vi "Increment Timer.vi"(8 "error in (no error)":errorcluster, 11 "Timer in":refnum<class "Timer.lvclass">) -> (0 "error out":errorcluster, 3 "Timer out":refnum<class "Timer.lvclass">)   [LabVIEW 2024, in "Timer.lvlib" / "Timer.lvclass"]
uses:
  Timer.lvclass
  Applications/National Instruments/LabVIEW 2024 64-bit/vi.lib/ActorFramework/Actor/Actor.lvclass
  Timer.lvclass/Timer.ctl
  <vilib>/ActorFramework/Actor/Actor.lvclass/Actor.ctl
  <vilib>/ActorFramework/Message Enqueuer/Message Enqueuer.lvclass/Message Enqueuer.ctl
  <vilib>/ActorFramework/Message Enqueuer/Init from Existing Queue.vi
  <vilib>/ActorFramework/Message Enqueuer/Enqueue.vi
  Timer Messages/Publish Updates Msg/Publish Updates Msg.lvclass
  Applications/National Instruments/LabVIEW 2024 64-bit/vi.lib/ActorFramework/Message/Message.lvclass
  Timer Messages/Stop Timer Msg/Stop Timer Msg.lvclass
  Timer Messages/Increment Timer Msg/Increment Timer Msg.lvclass
  <vilib>/ActorFramework/Message Priority Queue/Priority Enqueue.vi
  <vilib>/ActorFramework/Message Enqueuer/Message Enqueuer.lvclass
  <vilib>/ActorFramework/Actor/Actor.lvclass
  Users/elijahkerry/challenge-of-champions/Timer/Timer/Timer.lvclass
panel:
  out "x-y":dbl format="%#_6f"
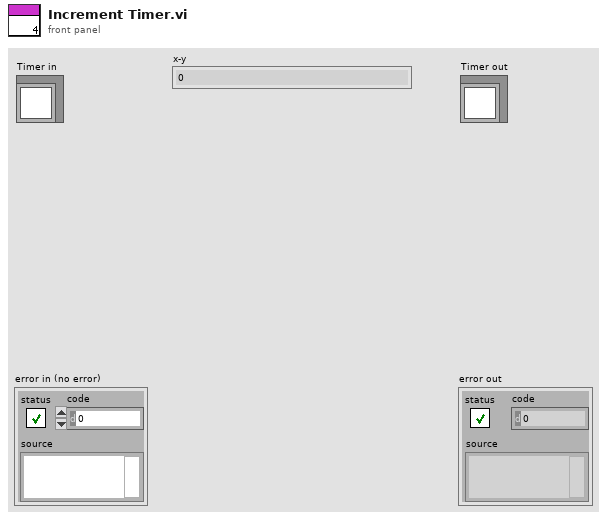
[diagram p1: front panel]
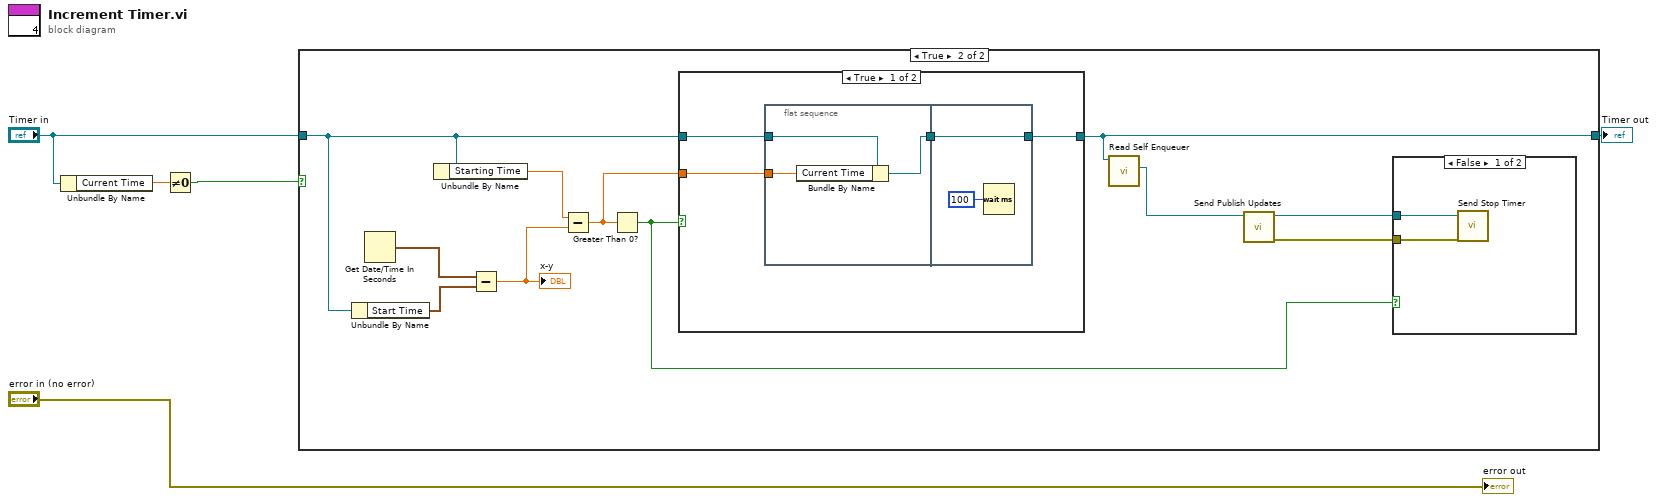
[diagram p0: block diagram]
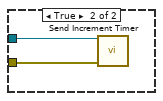
[diagram p3: hidden frame]
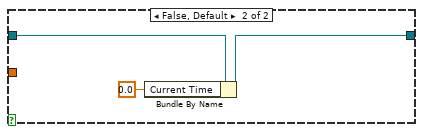
[diagram p4: hidden frame]
diagram:
  n1 = Unbundle By Name("Timer in") -> ("Current Time"=w3:dbl)
  n2 = Not Equal To 0?(x=w3) -> (x != 0?=w2:bool)
  n3 = case shown="True" w2 {
    tunnel: [w6 w9] -> w5
    tunnel: "Timer in" -> [w6 w10]
    frame False {
    }
    frame True {
      n4 = Unbundle By Name(w10) -> ("Start Time"=w14:timestamp)
      n5 = Get Date/Time In Seconds() -> (seconds since 1Jan1904=w13:timestamp)
      n6 = Unbundle By Name(w10) -> ("Starting Time"=w12:dbl)
      n7 = Subtract(x=w13, y=w14) -> (x-y=w11:dbl)
      "x-y" <- w11
      n8 = Subtract(x=w12, y=w11) -> (x-y=w8:dbl)
      n9 = Greater Than 0?(x=w8) -> (x > 0?=w7:bool)
      n10 = case shown="True" w7 {
        tunnel: w10 -> [w24 w33]
        tunnel: w8 -> [w23 _]
        tunnel: [w22 w32] -> w9
        frame True {
          n11 = flat-sequence {
            tunnel: w24 -> [w27]
            tunnel: w23 -> [w28]
            tunnel: [w26] -> w25
            tunnel: [w30] -> w22
            tunnel: w25 -> [w30]
            frame #0 {
              n12 = Bundle By Name(cluster=w27, "Current Time"=w28) -> (w26:refnum<class "Timer.lvclass">)
            }
            frame #1 {
              n13 = Wait (ms)(milliseconds to wait=u32 100) -> ()  [unwired: 1 out]
            }
          }
        }
        frame False, Default {
          n14 = Bundle By Name(cluster=w33, "Current Time"=0.0) -> (w32:refnum<class "Timer.lvclass">)
        }
      }
      n15 = call <vilib>:"Read Self Enqueuer.vi"("Actor"=w9) -> ("Self Enqueuer"=w17:refnum<class "Message Enqueuer.lvclass">)  [unwired: 10 in]
      n16 = call "Send Publish Updates.vi"("Message Enqueuer"=w17) -> ("error out"=w15:errorcluster, "Message Enqueuer out"=w16:refnum<class "Message Enqueuer.lvclass">)  [unwired: 9 in]
      n17 = case shown="False" w7 {
        tunnel: w16 -> [w19 w21]
        tunnel: w15 -> [w18 w20]
        frame False {
          n18 = call "Send Stop Timer.vi"("error in (no error)"=w18, "Message Enqueuer"=w19) -> ()  [unwired: 8 in, 2 out]
        }
        frame True {
          n19 = call "Send Increment Timer.vi"("error in (no error)"=w20, "Message Enqueuer"=w21) -> ()  [unwired: 8 in, 2 out]
        }
      }
    }
  }
  "Timer out" <- w5
  "error out" <- "error in (no error)"
